vi "Ctor.vi"(8 "error in (no error)":errorcluster, 11 "2DPanelBlank in":refnum<class "2DPanelBlank.lvclass">) -> (0 "error out":errorcluster, 3 "2DPanelBlank out":refnum<class "2DPanelBlank.lvclass">)   [LabVIEW 2020, in "OOPanel.lvlib" / "2DPanelBlank.lvclass"]
uses:
  2DPanelBlank.lvclass
  ArrayPanel/ArrayPanel.lvclass
  2D Index.ctl
  OOPanel.lvlib
  State.ctl
  Info.ctl
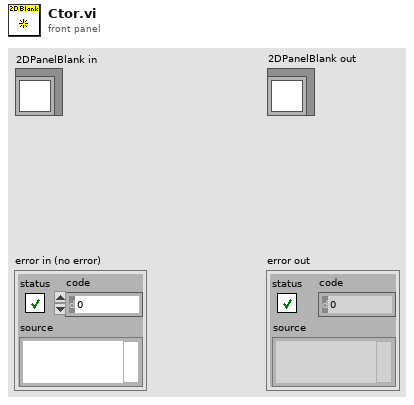
[diagram p1: front panel]
types:
  T1 = typedef "OOPanel.lvlib/2DPanelBlank.lvclass/Info.ctl" = cluster{"Index":T2, "State":T3, "Pull Count":i32}
  T2 = typedef "OOPanel.lvlib/2D Index.ctl" = cluster{"Row":i32, "Col":i32}
  T3 = typedef "OOPanel.lvlib/2DPanelBlank.lvclass/State.ctl" = enum16{"New", "Idle", "Pool", "Used", "No SP"}
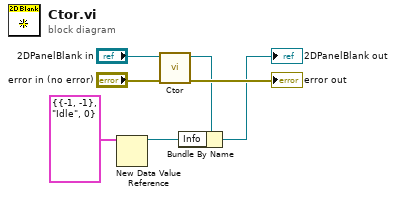
[diagram p0: block diagram]
diagram:
  n1 = New Data Value Reference(data value=T1 {"Index"={"Row"=-1, "Col"=-1}, "State"=enum."Idle", "Pull Count"=0} ("Info")) -> (data value reference=w1:refnum<data-value>)  [unwired: 1 in, 1 out]
  n2 = call-parent "Ctor.vi"("error in (no error)"="error in (no error)", "ArrayPanel in"="2DPanelBlank in") -> ("error out"=→"error out":errorcluster, "ArrayPanel out"=w3:refnum<class "2DPanelBlank.lvclass">)  [unwired: 8 in]
  n3 = Bundle By Name(cluster=w3, "Info"=w1) -> (→"2DPanelBlank out":refnum<class "2DPanelBlank.lvclass">)
